vi "UI Top Level.vi"(8 "error in":errorcluster) -> (0 "error out":errorcluster)   [LabVIEW 2020, in "UI.lvlib"]
uses:
  UI.lvlib
  Private Controls/Module Action.ctl
  Controller/Public Controls/IP Stats.ctl
  Private Controls/TabTools.ctl
  Public Controls/Module Data Cluster.ctl
  Public Controls/Config.ctl
  Controller/Public Controls/Config.ctl
  Private Controls/UI Action.ctl
  55c70144-0a05-4fb8-b549-1f89b1e31343.vi
  b2557411-5cff-4c84-9b89-16ab07a25453.vi
  27c827a8-6ce2-46ff-b742-8397f53ceddc.vi
  c3b89c2c-9874-4e6b-bcc8-0eccc53797a4.vi
  39dfc7b4-4df3-4aff-b378-9127056ea6e9.vi
  16cb41ff-8f3c-4f22-bc48-50ffacbfc1d7.vi
  075bdf41-c59e-4d84-85d6-4d97901147de.vi
  <vilib>/Utility/error.llb/Clear Errors.vi
  Controller/Controller.lvlib
  Architecture Support/Architecture Support.lvlib
  Error Handler/Error Handler.lvlib
panel:
  in  "Stop Search":bool
  in  "Local":bool
  in  "Search IP":string
  in  "Search":bool
  in  "Intro Screen":enum32{"Intro Screen"}(tab)
  out "User tools":T1=enum."Start"
  out "Searched:":string
  out "Address Responses":T2[](array[typedef])
  in  "Stop":bool
  out "Action":T3
  # "Welcome to NetScan\n\nBasic Functionality:\n- Enter an IP Address\n- Search for address on the local network\n- Conduct analysis into local devices\n\nProject Repo:\nhttps://github.com/aa-w/NetScan"
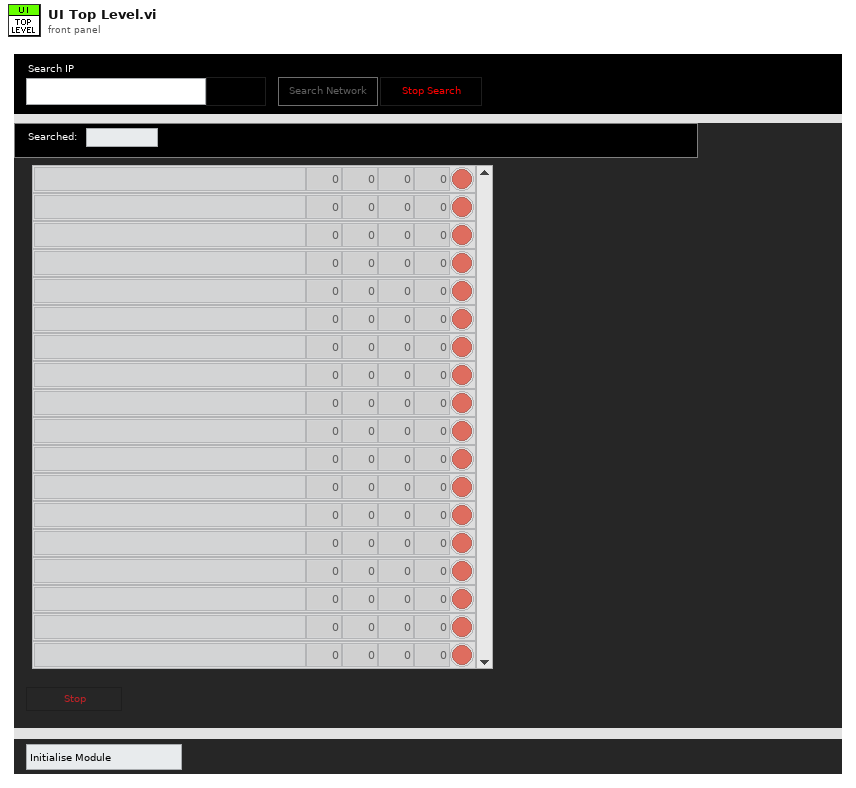
[diagram p1: front panel]
types:
  T1 = typedef "UI.lvlib/TabTools.ctl" = enum32{"Intro", "Start", "Search Tools", "Analysis Tools"}
  T2 = typedef "UI.lvlib/IP Stats.ctl" = cluster{"Address":string, "Average Response Time":i32, "Loss %":dbl, "Min Response Time":dbl, "Max Response Time":dbl, "Boolean":bool}
  T3 = typedef "UI.lvlib/Module Action.ctl" = enum16{"Initialise Module", "Connect", "Setup", "Pause", "Start", "Search", "Set IP", "Count Call", "Update UI", "Stop", "Post Results", "Wait: Time Elapsed", "Error", "Exit"}
  T4 = typedef "UI.lvlib/Module Data Cluster.ctl" = cluster{"Pause?":bool, "Iteration":i32, "Time Elapsed?":bool, "Config":T5, "Controller Config":T6, "Addresses Searched":i32}
  T5 = typedef "UI.lvlib/Config.ctl" = cluster{"Value":dbl}
  T6 = typedef "Controller.lvlib/Config.ctl" = cluster{"Value":dbl}
  T7 = typedef "UI.lvlib/UI Action.ctl" = enum16{"Intro", "Start", "Searching", "Analysis"}
  T8 = enum8{"Enabled", "Disabled", "Disabled and Grayed Out"}
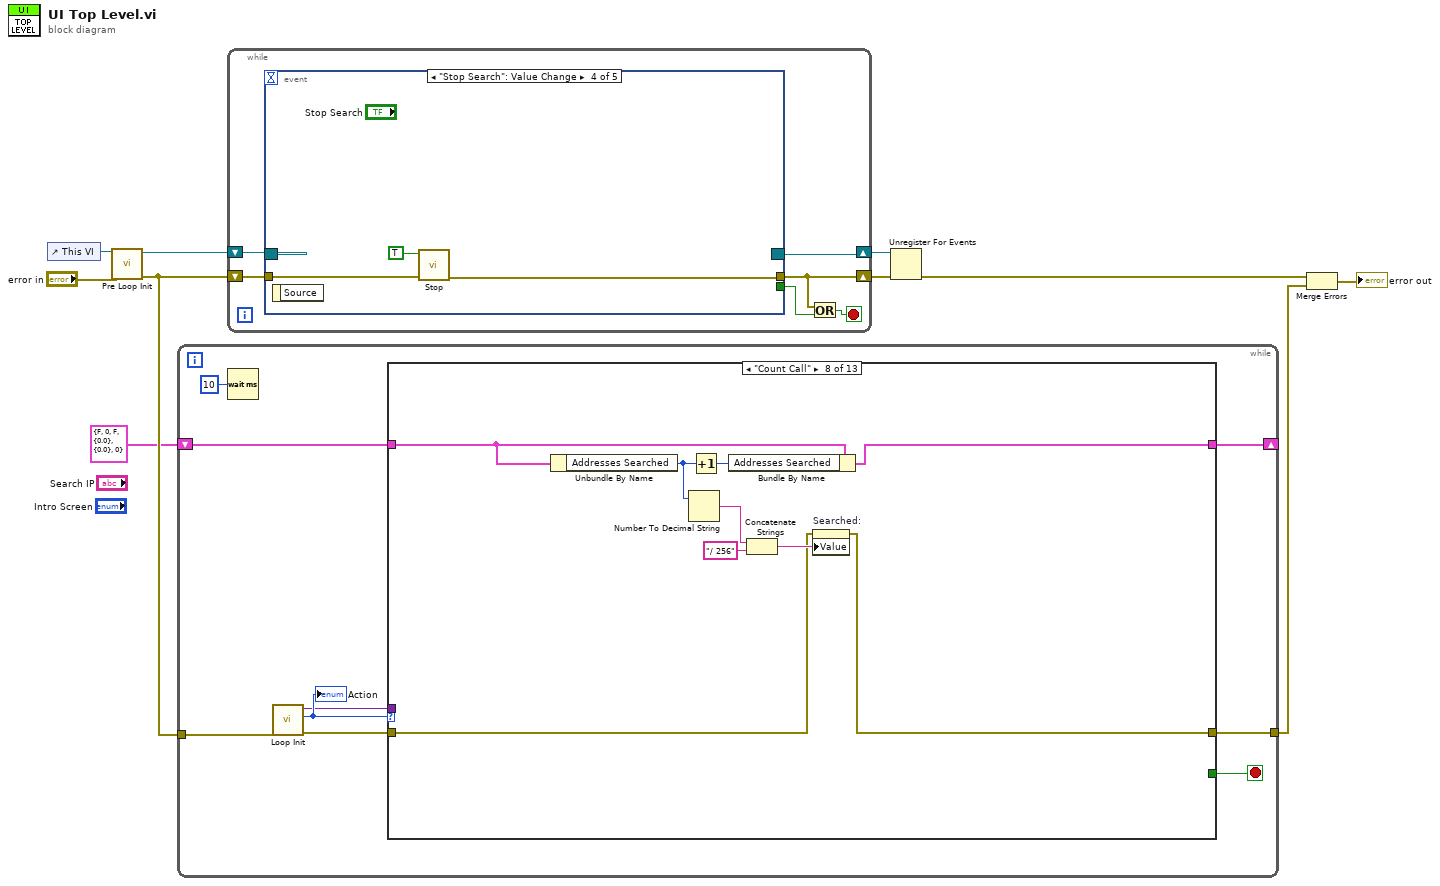
[diagram p0: block diagram]
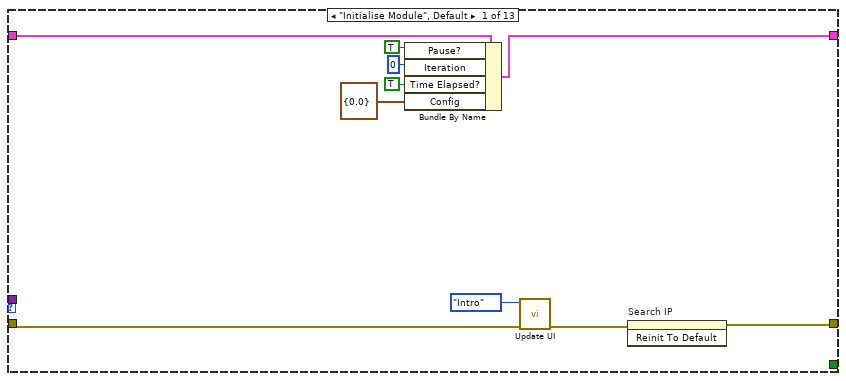
[diagram p2: hidden frame]
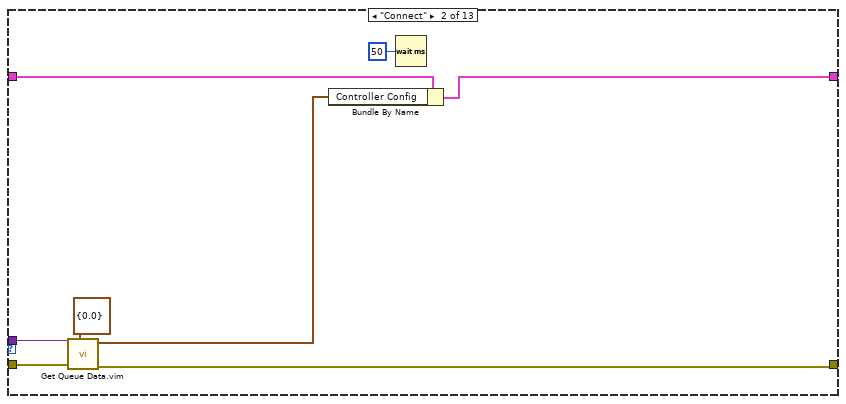
[diagram p3: hidden frame]
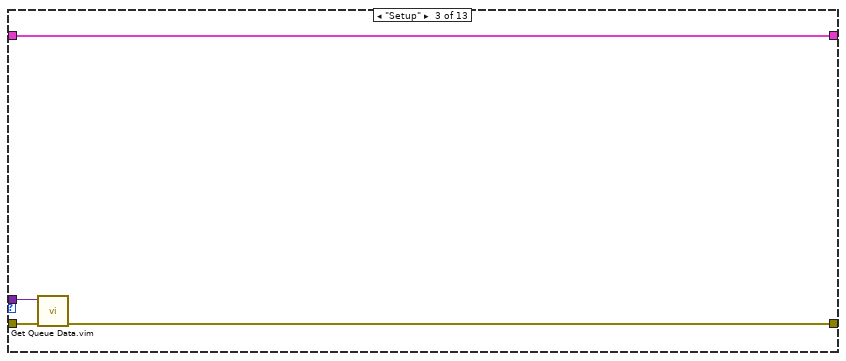
[diagram p4: hidden frame]
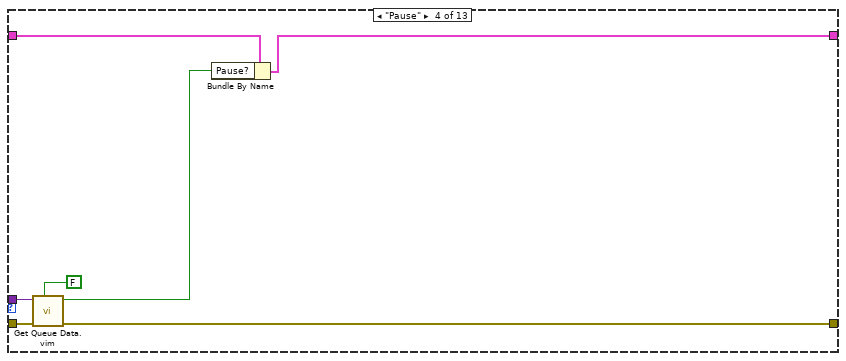
[diagram p5: hidden frame]
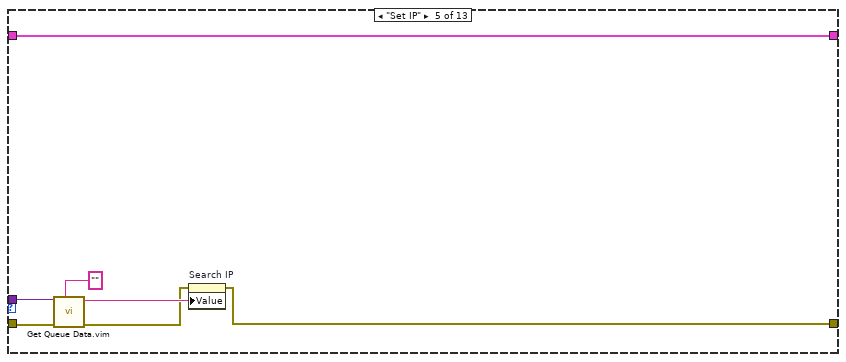
[diagram p6: hidden frame]
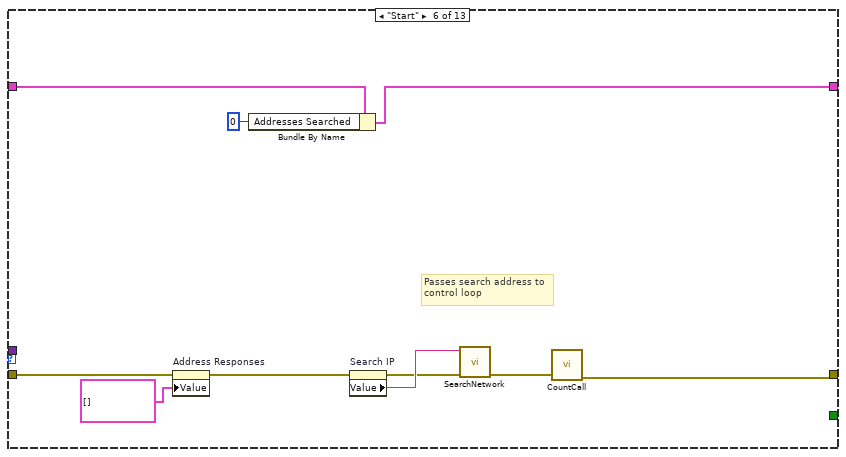
[diagram p7: hidden frame]
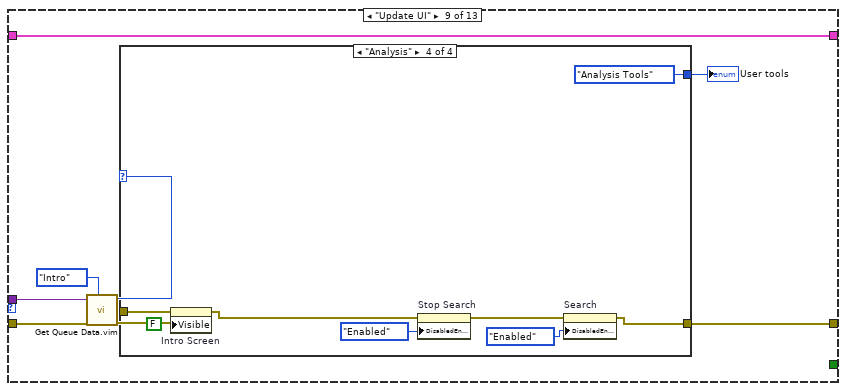
[diagram p9: hidden frame]
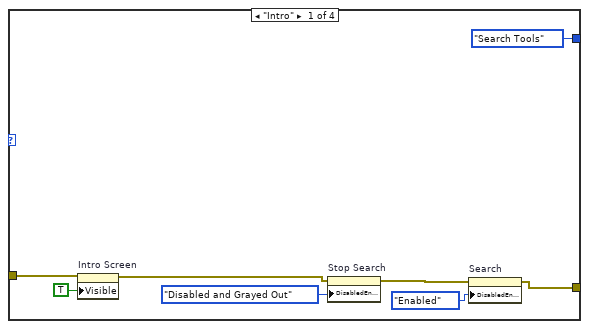
[diagram p10: hidden frame]
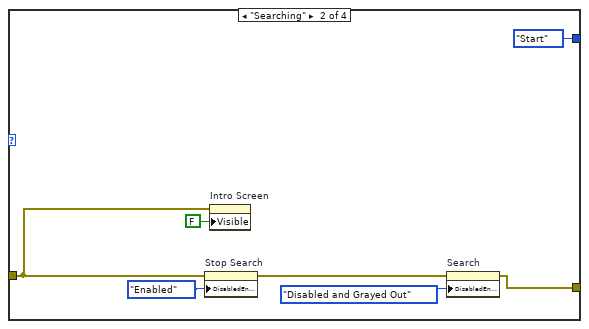
[diagram p11: hidden frame]
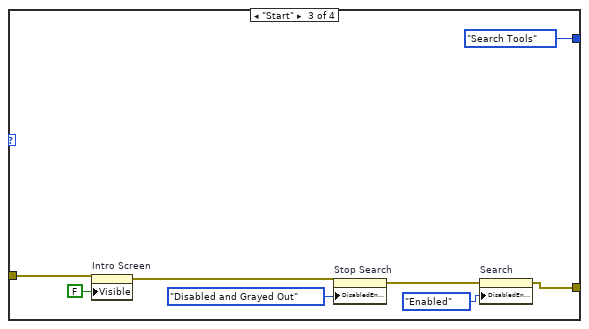
[diagram p12: hidden frame]
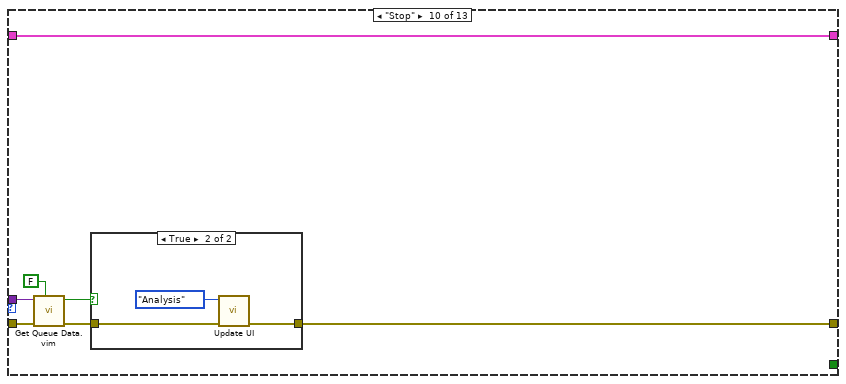
[diagram p13: hidden frame]
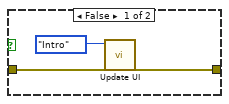
[diagram p14: hidden frame]
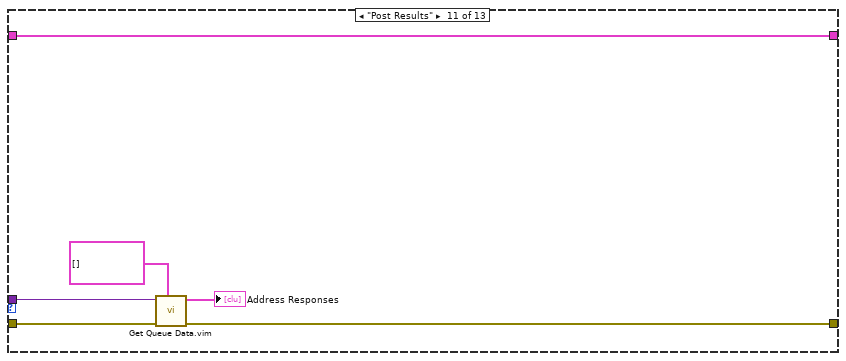
[diagram p15: hidden frame]
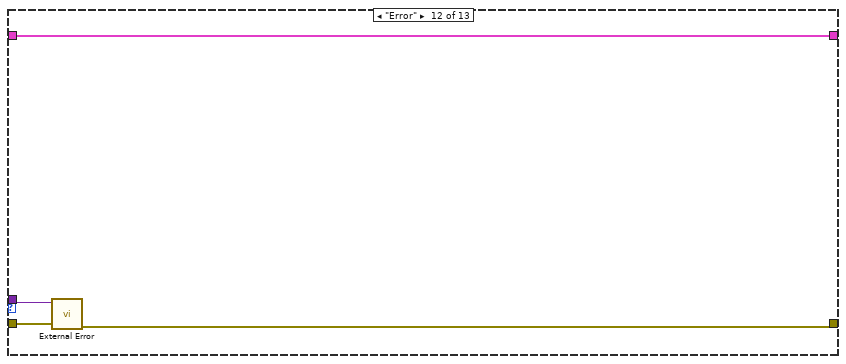
[diagram p16: hidden frame]
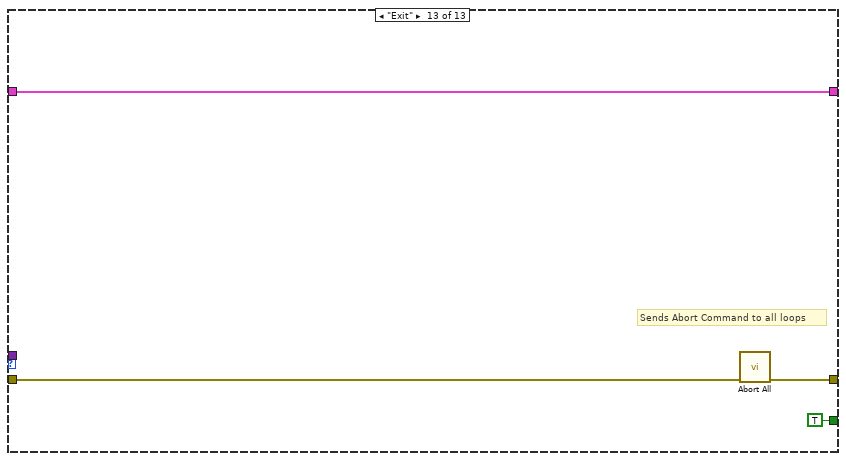
[diagram p17: hidden frame]
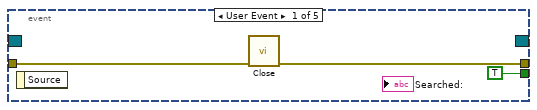
[diagram p18: hidden frame]
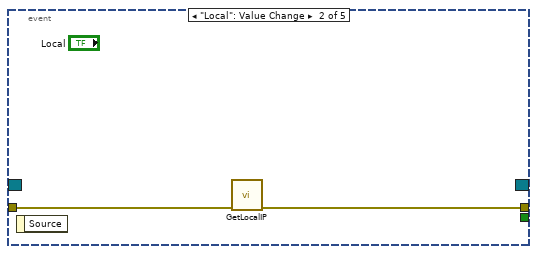
[diagram p19: hidden frame]
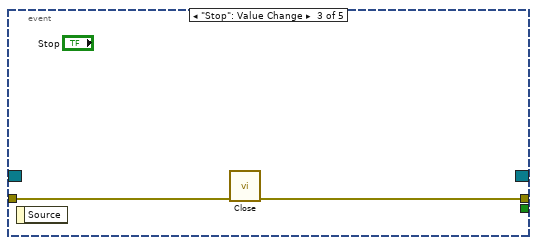
[diagram p20: hidden frame]
diagram:
  n1 = control-ref of="This VI"() -> (w4:refnum<vi>)
  n2 = call "Pre Loop Init.vi"("error in (no error)"="error in", "Ref In"=w4) -> ("error out"=w7:errorcluster, "Event Registration Refnum"=w6:refnum<event-registration>)  [unwired: 8 in]
  n3 = while {
    shift-right: [w11] -> _
    shift-left: T4 {"Pause?"=FALSE, "Iteration"=0, "Time Elapsed?"=FALSE, "Config"={"Value"=0.0}, "Controller Config"={"Value"=0.0}, "Addresses Searched"=0} ("Module Data Cluster") -> [w12]
    tunnel: w7 -> [w18]
    tunnel: [w15] -> w8
    stop <- w14 stop-if-true
    n4 = Wait (ms)(milliseconds to wait=u32 10) -> ()  [unwired: 1 out]
    n5 = call "Loop Init.vi"("error in (no error)"=w18) -> ("error out"=w16:errorcluster, "Action"=w17:T3, "Data"=w13:variant)  [unwired: 8 in]
    "Action" <- w17
    n6 = case shown="\"Count Call\"" w17 {
      tunnel: w16 -> [w20 w37 w41 w48 w53 w57 w66 w69 w84 w122 w134 w137 w140]
      tunnel: [w23 w36 w40 w46 w55 w59 w66 w68 w78 w118 w131 w135 w139] -> w15
      tunnel: [w29 w31 w38 w43 w54 w65 w67 w76 w80 w120 w130 w138 w141] -> w11
      tunnel: [_ _ _ _ _ _ _ _ _ _ _ _ TRUE] -> w14
      tunnel: w13 -> [_ w35 w39 w47 w52 _ _ _ w83 w121 w133 w136 _]
      tunnel: w12 -> [w24 w32 w38 w42 w54 w64 w67 w75 w80 w120 w130 w138 w141]
      frame "Initialise Module", Default {
        n7 = Bundle By Name(cluster=w24, "Pause?"=TRUE, "Iteration"=0, "Time Elapsed?"=TRUE, "Config"=T5 {"Value"=0.0}) -> (w29:T4)
        n8 = call "Update UI.vi"("error in (no error)"=w20, "Data"=UI_Action."Intro" ("Action")) -> ("error out"=w22:errorcluster)  [unwired: 9 in]
        n9 = invoke on="Search IP" class="Str" method="Reinit To Default"(error in=w22) -> (error out=w23:errorcluster)  [unwired: 2 in, 2 out]
      }
      frame "Connect" {
        n10 = call "Get Queue Data.vim"("Default Value"=T6 {"Value"=0.0} ("Config"), "error in"=w37, "Variant"=w35) -> ("error out"=w36:errorcluster, "Module Data"=w33:T6)  [unwired: 7 in]
        n11 = Bundle By Name(cluster=w32, "Controller Config"=w33) -> (w31:T4)
        n12 = Wait (ms)(milliseconds to wait=u32 50) -> ()  [unwired: 1 out]
      }
      frame "Setup" {
        n13 = call "Get Queue Data.vim"("error in"=w41, "Variant"=w39) -> ("error out"=w40:errorcluster)  [unwired: 8 in, 1 out]
      }
      frame "Pause" {
        n14 = call "Get Queue Data.vim"("Default Value"=FALSE, "error in"=w48, "Variant"=w47) -> ("error out"=w46:errorcluster, "Module Data"=w44:bool)  [unwired: 7 in]
        n15 = Bundle By Name(cluster=w42, "Pause?"=w44) -> (w43:T4)
      }
      frame "Set IP" {
        n16 = call "Get Queue Data.vim"("Default Value"="", "error in"=w53, "Variant"=w52) -> ("error out"=w49:errorcluster, "Module Data"=w50:string)  [unwired: 7 in]
        n17 = property on="Search IP" class="Str"(error in=w49, "Value"=w50) -> (error out=w55:errorcluster)  [unwired: 1 in, 1 out]
      }
      frame "Start" {
        # "Passes search address to\ncontrol loop"
        n18 = property on="Address Responses" class="Arr (strict)"(error in=w57, "Value"=T2[] [] ("Address Responses")) -> (error out=w56:errorcluster)  [unwired: 1 in, 1 out]
        n19 = Bundle By Name(cluster=w64, "Addresses Searched"=0) -> (w65:T4)
        n20 = property on="Search IP" class="Str"(error in=w56) -> (error out=w61:errorcluster, "Value"=w62:string)  [unwired: 1 in, 1 out]
        n21 = call "SearchNetwork.vi"("error in (no error)"=w61, "Data"=w62) -> ("error out"=w60:errorcluster)  [unwired: 9 in]
        n22 = call "CountCall.vi"("error in (no error)"=w60) -> ("error out"=w59:errorcluster)  [unwired: 10 in]
      }
      frame "Search" {
      }
      frame "Count Call" {
        n23 = Unbundle By Name(w75) -> ("Addresses Searched"=w73:i32)
        n24 = Number To Decimal String(number=w73) -> (decimal integer string=w70:string)  [unwired: 1 in]
        n25 = Increment(x=w73) -> (x+1=w74:i32)
        n26 = Bundle By Name(cluster=w75, "Addresses Searched"=w74) -> (w76:T4)
        n27 = Concatenate Strings(w70, "/ 256" ("string")) -> (w71:string)
        n28 = property on="Searched:" class="Str"(error in=w69, "Value"=w71) -> (error out=w68:errorcluster)  [unwired: 1 in, 1 out]
      }
      frame "Update UI" {
        n29 = call "Get Queue Data.vim"("Default Value"=UI_Action."Intro" ("Action"), "error in"=w84, "Variant"=w83) -> ("error out"=w79:errorcluster, "Module Data"=w81:T7)  [unwired: 7 in]
        n30 = case shown="\"Analysis\"" w81 {
          tunnel: w79 -> [w90 w93 w105 w113]
          tunnel: [w85 w96 w100 w108] -> w78
          tunnel: [TabTools."Search Tools" ("User tools") TabTools."Start" ("User tools") TabTools."Search Tools" ("User tools") TabTools."Analysis Tools" ("User tools")] -> w77
          frame "Intro" {
            n31 = property on="Intro Screen" class="TabCtl (strict)"(error in=w90, "Visible"=TRUE) -> (error out=w86:errorcluster)  [unwired: 1 in, 1 out]
            n32 = property on="Stop Search" class="Bool"(error in=w86, "DisabledEnum"=T8."Disabled and Grayed Out" ("Disabled")) -> (error out=w89:errorcluster)  [unwired: 1 in, 1 out]
            n33 = property on="Search" class="Bool"(error in=w89, "DisabledEnum"=T8."Enabled" ("Disabled")) -> (error out=w85:errorcluster)  [unwired: 1 in, 1 out]
          }
          frame "Searching" {
            n34 = property on="Stop Search" class="Bool"(error in=w93, "DisabledEnum"=T8."Enabled" ("Disabled")) -> (error out=w97:errorcluster)  [unwired: 1 in, 1 out]
            n35 = property on="Intro Screen" class="TabCtl (strict)"(error in=w93, "Visible"=FALSE) -> ()  [unwired: 1 in, 2 out]
            n36 = property on="Search" class="Bool"(error in=w97, "DisabledEnum"=T8."Disabled and Grayed Out" ("Disabled")) -> (error out=w96:errorcluster)  [unwired: 1 in, 1 out]
          }
          frame "Start" {
            n37 = property on="Intro Screen" class="TabCtl (strict)"(error in=w105, "Visible"=FALSE) -> (error out=w103:errorcluster)  [unwired: 1 in, 1 out]
            n38 = property on="Stop Search" class="Bool"(error in=w103, "DisabledEnum"=T8."Disabled and Grayed Out" ("Disabled")) -> (error out=w101:errorcluster)  [unwired: 1 in, 1 out]
            n39 = property on="Search" class="Bool"(error in=w101, "DisabledEnum"=T8."Enabled" ("Disabled")) -> (error out=w100:errorcluster)  [unwired: 1 in, 1 out]
          }
          frame "Analysis" {
            n40 = property on="Intro Screen" class="TabCtl (strict)"(error in=w113, "Visible"=FALSE) -> (error out=w109:errorcluster)  [unwired: 1 in, 1 out]
            n41 = property on="Stop Search" class="Bool"(error in=w109, "DisabledEnum"=T8."Enabled" ("Disabled")) -> (error out=w112:errorcluster)  [unwired: 1 in, 1 out]
            n42 = property on="Search" class="Bool"(error in=w112, "DisabledEnum"=T8."Enabled" ("Disabled")) -> (error out=w108:errorcluster)  [unwired: 1 in, 1 out]
          }
        }
        "User tools" <- w77
      }
      frame "Stop" {
        n43 = call "Get Queue Data.vim"("Default Value"=FALSE, "error in"=w122, "Variant"=w121) -> ("error out"=w119:errorcluster, "Module Data"=w116:bool)  [unwired: 7 in]
        n44 = case shown="True" w116 {
          tunnel: w119 -> [w124 w127]
          tunnel: [w123 w126] -> w118
          frame False {
            n45 = call "Update UI.vi"("error in (no error)"=w124, "Data"=UI_Action."Intro" ("Action")) -> ("error out"=w123:errorcluster)  [unwired: 9 in]
          }
          frame True {
            n46 = call "Update UI.vi"("error in (no error)"=w127, "Data"=UI_Action."Analysis" ("Action")) -> ("error out"=w126:errorcluster)  [unwired: 9 in]
          }
        }
      }
      frame "Post Results" {
        n47 = call "Get Queue Data.vim"("Default Value"=T2[] [] ("Response Array"), "error in"=w134, "Variant"=w133) -> ("error out"=w131:errorcluster, "Module Data"=→"Address Responses":T2[])  [unwired: 7 in]
      }
      frame "Error" {
        n48 = call "External Error.vi"("error in (no error)"=w137, "Data"=w136) -> ("error out"=w135:errorcluster)  [unwired: 9 in]
      }
      frame "Exit" {
        # "Sends Abort Command to all loops"
        n49 = call "Abort All.vi"("error in (no error)"=w140) -> ("error out"=w139:errorcluster)  [unwired: 10 in]
      }
    }
  }
  n50 = while {
    shift-right: [w145] -> w10
    shift-left: w7 -> [w144]
    shift-right: [w147] -> w5
    shift-left: w6 -> [w148]
    stop <- w146 stop-if-true
    n51 = event shown="[3] \"Stop Search\": Value Change" {
      selector: w148 -> [_ _ _ _ _]
      dyn-events: [_ _ _ _ _] -> w147
      timeout: _ -> [_ _ _ _ _]
      tunnel: [w150 w152 w154 w156 w159] -> w145
      tunnel: w144 -> [w151 w153 w155 w158 w162]
      tunnel: [TRUE _ _ _ _] -> w143
      event User Event {
        n52 = event-data() -> ()  [unwired: 1 in, 1 out]
        n53 = call "Close.vi"("error in (no error)"=w151) -> ("error out"=w150:errorcluster)  [unwired: 10 in]
      }
      event "Local": Value Change {
        n54 = event-data() -> ()  [unwired: 1 in, 1 out]
        n55 = call "GetLocalIP.vi"("error in (no error)"=w153) -> ("error out"=w152:errorcluster)  [unwired: 10 in]
      }
      event "Stop": Value Change {
        n56 = event-data() -> ()  [unwired: 1 in, 1 out]
        n57 = call "Close.vi"("error in (no error)"=w155) -> ("error out"=w154:errorcluster)  [unwired: 10 in]
      }
      event "Stop Search": Value Change {
        n58 = event-data() -> ()  [unwired: 1 in, 1 out]
        n59 = call "Stop.vi"("error in (no error)"=w158, "Data"=TRUE) -> ("error out"=w156:errorcluster)  [unwired: 9 in]
      }
      event "Search": Value Change {
        n60 = event-data() -> ()  [unwired: 1 in, 1 out]
        n61 = call "Start.vi"("error in (no error)"=w162) -> ("error out"=w160:errorcluster)  [unwired: 10 in]
        n62 = call "Update UI.vi"("error in (no error)"=w160, "Data"=UI_Action."Searching" ("Action")) -> ("error out"=w159:errorcluster)  [unwired: 9 in]
      }
    }
    n63 = Or(x=w145, y=w143) -> (x .or. y?=w146:bool)
  }
  n64 = Unregister For Events(event registration refnum=w5, error in=w10) -> (error out=w9:errorcluster)
  n65 = Merge Errors(w9, w8) -> (→"error out":errorcluster)
